vi "init.vi"(0 "Device Configuration Test in":refnum<class "Device Configuration Test.lvclass">, 1 "Unique ID Length":u8, 2 "TEDS Status Test":T1, 5 "error in (no error)":errorcluster, 6 "Test Scenario":T2, 7 "ILC":refnum<class "ILC.lvclass">, 8 "Signal Name":string, 9 "Log":refnum<class "ITestLog.lvclass">) -> (14 "Device Configuration Test out":refnum<class "Device Configuration Test.lvclass">, 19 "error out":errorcluster)   [LabVIEW 2015, in "Device Configuration Test.lvclass"]
uses:
  Device Configuration Test.lvclass
  Model/TestLog/ITestLog/ITestLog.lvclass
  Typedefs/TestScenarioTypes.ctl
  <userlib>/Common/ilc/ILC/ILC.lvclass
  Typedefs/1-Wire Test.ctl
  Device Configuration Test.lvclass/Device Configuration Test.ctl
  Typedefs/ILCBTTypedefs.lvlib
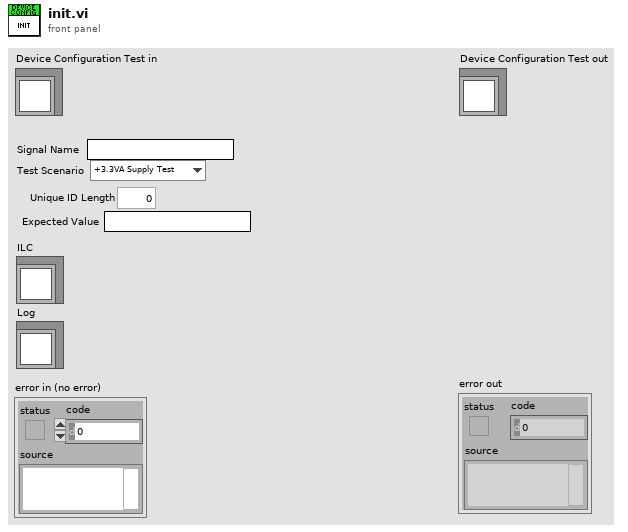
[diagram p1: front panel]
types:
  T1 = typedef "ILCBTTypedefs.lvlib/1-Wire Test.ctl" = cluster{"Expected Value":string}
  T2 = typedef "ILCBTTypedefs.lvlib/TestScenarioTypes.ctl" = enum16{"+3.3VA Supply Test", "+3.3VD Supply Test", "+5VA Supply Test", "+5VD Supply Test", "Unique ID Test", "TEDS Status Test", "LIMSW1_TTL Low Test", "LIMSW1_TTL High Test", "LIMSW2_TTL Low Test", "LIMSW2_TTL High Test", "Tachometer Test", "SSR_TTL Low Test", "SSR_TTL High Test", "SM_GPI Low Test", "SM_GPI High Test", "CW Motion Without Limit Test", "CW Motion With Limit Test", "CW Motion With Both Limits Test", "CW Motion on CCW Limit Test", "CCW Motion Without Limit Test", "CCW Motion With Limit Test", "CCW Motion With Both Limits Test", "CCW Motion on CW Limit Test", "RS232-TXD Low Test", "RS232-TXD High Test", "RS232-RTS Low Test", "RS232-RTS High Test", "RS232-RXD Low Test", "RS232-RXD High Test", "RS232-CTS Low Test", "RS232-CTS High Test", "Out_SS Low Test", "Out_SS High Test", "Out_SDI Low Test", "Out_SDI High Test", "Out_SCLK Low Test", "Out_SCLK High Test", "Reset Low Test", "Reset High Test", "1 Channel ADC Test", "3 Channel ADC Test", "5 Channel ADC Test", "Vref Test", "ROT Test", "DAC1 Test", "DAC2 Test", "DAC3 Test", "DAC4 Test", "BIAS Test", "EXC1 Test", "EXC2 Test", "EXC3 Test", "EXC4 Test"}
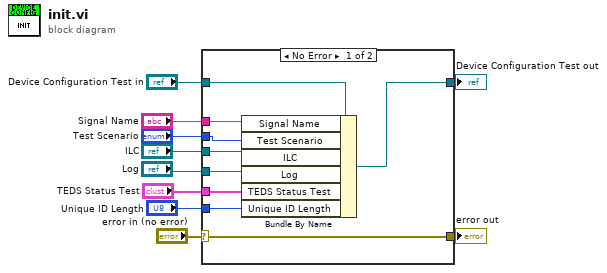
[diagram p0: block diagram]
diagram:
  n1 = case shown="No Error" "error in (no error)" {
    selector: "error in (no error)" -> [w19 w21]
    tunnel: [w19 w21] -> w9
    tunnel: [w15 w20] -> w7
    tunnel: "Device Configuration Test in" -> [w18 w20]
    tunnel: "Signal Name" -> [w14 _]
    tunnel: "Test Scenario" -> [w13 _]
    tunnel: "ILC" -> [w16 _]
    tunnel: "Log" -> [w17 _]
    tunnel: "TEDS Status Test" -> [w12 _]
    tunnel: "Unique ID Length" -> [w11 _]
    frame No Error {
      n2 = Bundle By Name(cluster=w18, "Signal Name"=w14, "Test Scenario"=w13, "ILC"=w16, "Log"=w17, "TEDS Status Test"=w12, "Unique ID Length"=w11) -> (w15:refnum<class "Device Configuration Test.lvclass">)
    }
    frame Error {
    }
  }
  "error out" <- w9
  "Device Configuration Test out" <- w7
